vi "Dynamixel XL320 Search Motors.vi"(4 "Ending ID (252)":u8=252, 5 "Search Timeout (10000 ms)":u32=10000, 6 "Starting ID (0)":u8, 7 "Force Baud Rate (True)":bool, 8 "error in (no error)":errorcluster, 10 "Baud rate (1,000,000 bps)":T1=3 items=["9600 bps", "57600 bps", "115200 bps", "1,000,000 bps"], 11 "VISA resource name":refnum<visa-resource-name>) -> (0 "error out":errorcluster, 2 "Motors IDs Found":u8[](array[numeric]))   [LabVIEW 2015]
uses:
  <instrlib>/Dynamixel XL320/Public/Motor Operation/Low Level/XL320_Baud Setting.ctl
  <instrlib>/Dynamixel XL320/Dynamixel XL320.lvlib
panel:
  out "Searching for motor":bool
  in  "Tab Control":enum32{"Port setup", "Auto-detect settings"}(tab)
  # "Ghislain REMY, IUT de Cachan, 2015 December 2015"
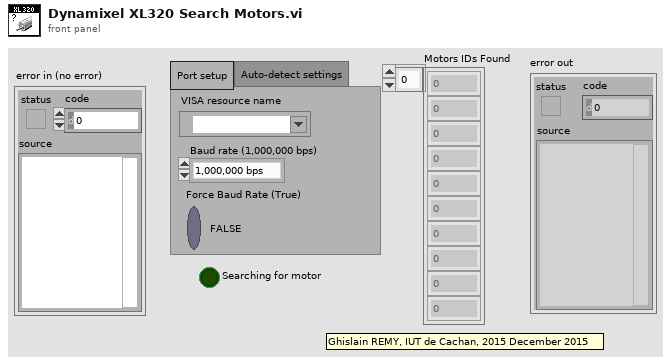
[diagram p1: front panel]
types:
  T1 = typedef "Dynamixel XL320.lvlib/XL320_Baud Setting.ctl" = u8
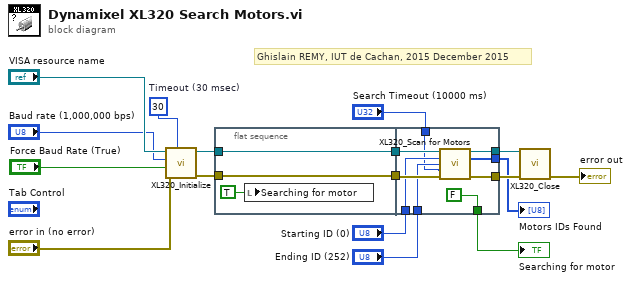
[diagram p0: block diagram]
diagram:
  w2 = u32 30  # Timeout (30 msec)
  # "Ghislain REMY, IUT de Cachan, 2015 December 2015"
  n1 = call <instrlib>:"XL320_Initialize.vi"("Timeout (30 msec)"=w2, "error in (no error)"="error in (no error)", "Force Baud Rate (True)"="Force Baud Rate (True)", "Baud rate (1,000,000 bps)"="Baud rate (1,000,000 bps)", "VISA resource name"="VISA resource name") -> ("error out"=w11:errorcluster, "VISA resource name out"=w12:refnum<visa-resource-name>)  [unwired: 5 in]
  n2 = flat-sequence {
    tunnel: w11 -> [w19]
    tunnel: w12 -> [w20]
    tunnel: [w20] -> w17
    tunnel: [w19] -> w16
    tunnel: [w27] -> w6
    tunnel: [w25] -> w5
    tunnel: [w26] -> w3
    tunnel: "Search Timeout (10000 ms)" -> [w21]
    tunnel: "Starting ID (0)" -> [w23]
    tunnel: "Ending ID (252)" -> [w22]
    tunnel: w17 -> [w28]
    tunnel: w16 -> [w24]
    tunnel: [FALSE ("Searching for motor")] -> w7
    frame #0 {
      n3 = local write "Searching for motor"(TRUE ("Searching for motor")) -> ()
    }
    frame #1 {
      n4 = call <instrlib>:"XL320_Scan for Motors.vi"("VISA resource name"=w28, "Starting ID (0)"=w23, "Ending ID (252)"=w22, "Search Timeout (10000 ms)"=w21, "error in (no error)"=w24) -> ("VISA resource name out"=w27:refnum<visa-resource-name>, "Motors IDs Found"=w26:u8[], "error out"=w25:errorcluster)  [unwired: 8 in]
    }
  }
  n5 = call <instrlib>:"XL320_Close.vi"("error in (no error)"=w5, "VISA resource name"=w6) -> ("error out"=→"error out":errorcluster)  [unwired: 9 in]
  "Searching for motor" <- w7
  "Motors IDs Found" <- w3
